vi "Application Settings Updated.vi"(8 "error in (no error)":errorcluster, 10 "Reply Payload":T1) -> (0 "error out":errorcluster)   [LabVIEW 2018, in "Settings Editor.lvlib"]
doc: "Request Settings Editor to return the latest settings. The Settings Editor can send the applications settings as a reply or via broadcast.\n_____\nCreated using Delacor QMH Event Scripter 4.1.0.75.\n_____\nBased on Delacor QMH Project Template 4.1.0.59."
uses:
  Settings Editor.lvlib
  Update Application Settings (Reply Payload)--cluster.ctl
  Settings--cluster.ctl
  Delacor/PPLs/CML_Shared.lvlibp/Signal Type--enum.ctl
  Delacor/PPLs/CML_Shared.lvlibp/Calibration Values--cluster.ctl
  Delacor/PPLs/CML_Shared.lvlibp
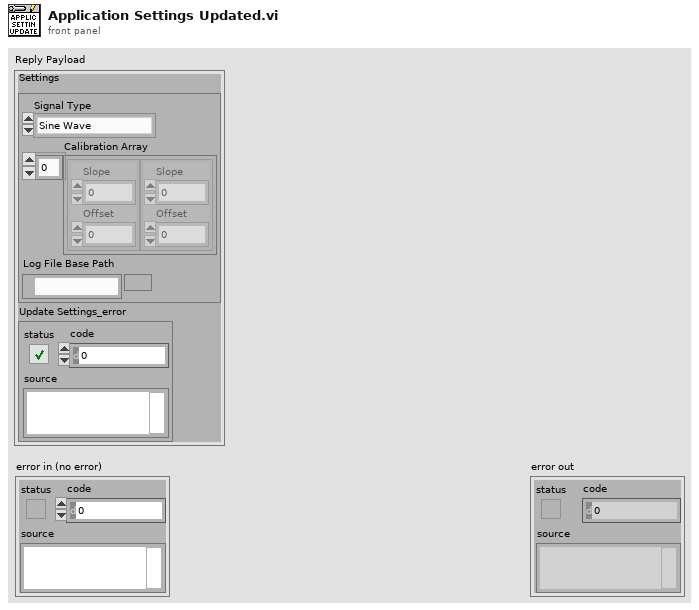
[diagram p1: front panel]
types:
  T1 = typedef "Settings Editor.lvlib/Update Application Settings (Reply Payload)--cluster.ctl" = cluster{"Settings":T2, "Update Settings_error":errorcluster}
  T2 = typedef "Settings Editor.lvlib/Settings--cluster.ctl" = cluster{"Signal Type":T3, "Calibration Array":T4[], "Log File Base Path":path}
  T3 = typedef "CML_Shared.lvlibp/Signal Type--enum.ctl" = enum16{"Sine Wave", "Square with Noise"}
  T4 = typedef "CML_Shared.lvlibp/Calibration Values--cluster.ctl" = cluster{"Slope":dbl, "Offset":dbl}
  T5 = typedef "Settings Editor.lvlib/Broadcast Events--cluster.ctl" = cluster{"Module Did Init":refnum<user-event>, "Status Updated":refnum<user-event>, "Error Reported":refnum<user-event>, "Module Did Stop":refnum<user-event>, "Update Module Execution Status":refnum<user-event>, "Application Settings Updated":refnum<user-event>}
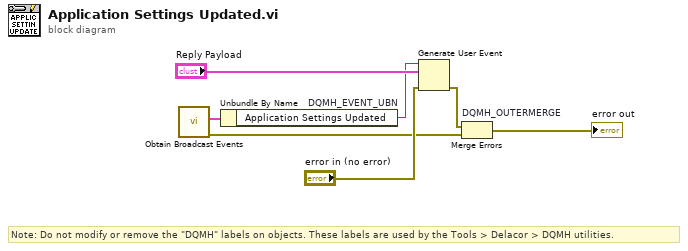
[diagram p0: block diagram]
diagram:
  # "Note: Do not modify or remove the \"DQMH\" labels on objects. These labels are used by the Tools > Delacor > DQMH utilities."
  n1 = call "Obtain Broadcast Events.vi"() -> ("error out"=w2:errorcluster, "Settings Editor Broadcast Events"=w1:T5)  [unwired: 10 in]
  n2 = Unbundle By Name "DQMH_EVENT_UBN"(w1) -> ("Application Settings Updated"=w4:refnum<user-event>)
  n3 = Generate User Event(user event=w4, event data cluster="Reply Payload", error in="error in (no error)") -> (error out=w3:errorcluster)  [unwired: 1 in, 1 out]
  n4 = Merge Errors "DQMH_OUTERMERGE"(w3, w2) -> (→"error out":errorcluster)
